vi "datosLecturaQR_to_Arduino.vi"(8 "error in (no error)":errorcluster, 9 "LECTURA QR INPUT":T1={"COORD X"=0, "COORD  Y"=0, "NºASICS"=1, "SELECCIÓN DE BANDEJA"=enum."BANDEJA ENTRADA", "CONTEO QR"=0}, 11 "VISA resource name":refnum<visa-resource-name>) -> (0 "error IO":errorcluster, 2 "celda de comienzo leída":string)   [LabVIEW 2019]
uses:
  TYPE'S DEF/INPUT LECTURA_QR.ctl
  <vilib>/Utility/error.llb/Error Cluster From Error Code.vi
  <vilib>/ErrorRing/Error Ring.xnode
panel:
  out "trama datos":string
  # "CELDA DE COMIENZO"
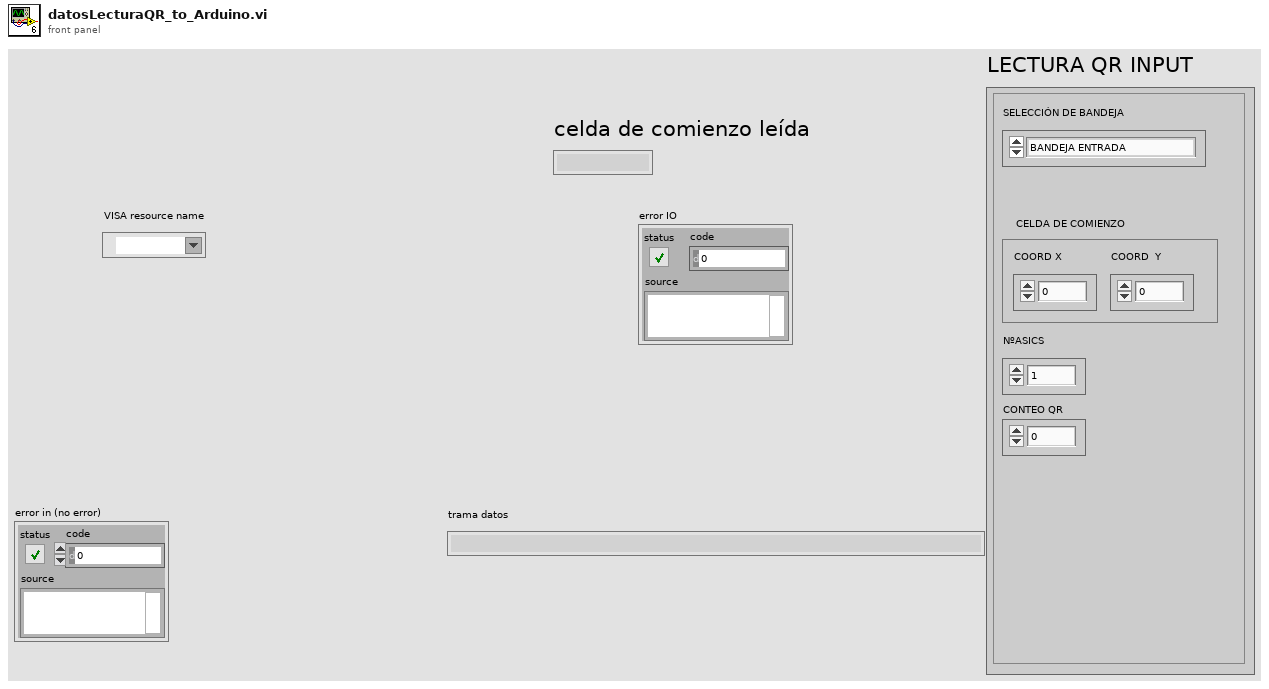
[diagram p1: front panel]
types:
  T1 = typedef "INPUT LECTURA_QR.ctl" = cluster{"COORD X":u16, "COORD  Y":u16, "NºASICS":u32, "SELECCIÓN DE BANDEJA":enum16{"BANDEJA ENTRADA", "BANDEJA OK", "BANDEJA NOK"}, "CONTEO QR":u32}
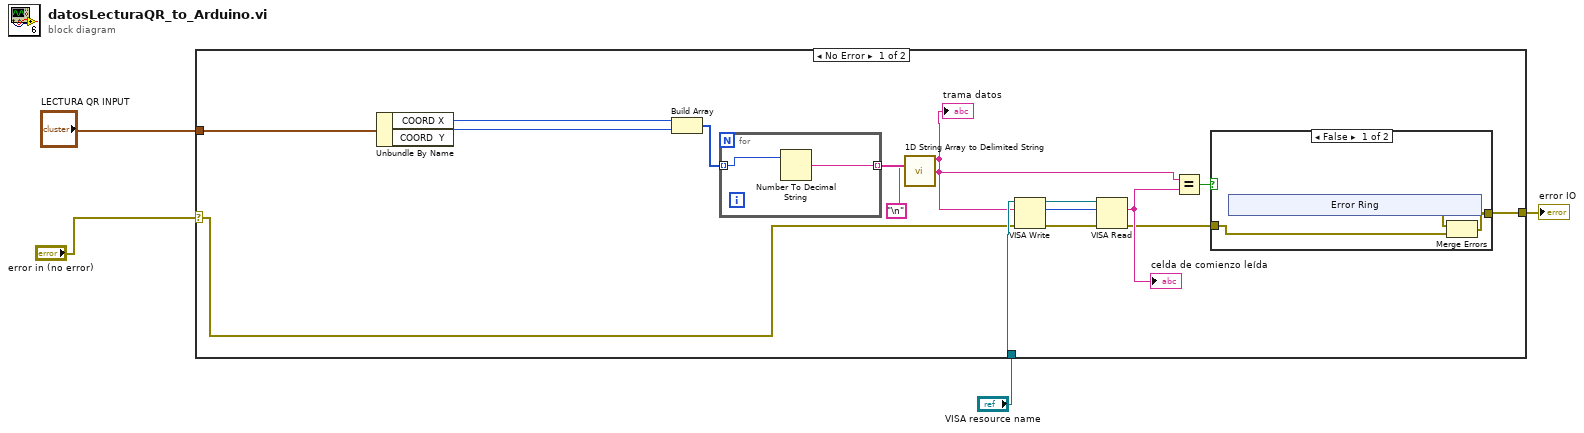
[diagram p0: block diagram]
diagram:
  n1 = case shown="No Error" "error in (no error)" {
    selector: "error in (no error)" -> [w16 w32]
    tunnel: "VISA resource name" -> [w17 _]
    tunnel: [w9 w32] -> w2
    tunnel: "LECTURA QR INPUT" -> [w5 _]
    frame No Error {
      n2 = Unbundle By Name(w5) -> ("COORD X"=w7:u16, "COORD  Y"=w6:u16)
      n3 = Build Array(w7, w6) -> (w20:u16[])
      n4 = for {
        tunnel: w20 -> [w30] mode=indexing
        tunnel: [w31] -> w19 mode=indexing
        n5 = Number To Decimal String(number=w30) -> (decimal integer string=w31:string)  [unwired: 1 in]
      }
      n6 = call <vilib>:"1D String Array to Delimited String.vi"("delimiter"="\n", "string array"=w19) -> ("delimited string"=w12:string)  [unwired: 9 in]
      "trama datos" <- w12
      n7 = VISA Write(VISA resource name=w17, write buffer=w12, error in (no error)=w16) -> (VISA resource name out=w14:refnum<visa-resource-name>, return count=w13:u32, error out=w15:errorcluster)
      n8 = VISA Read(VISA resource name=w14, byte count=w13, error in (no error)=w15) -> (read buffer=w11:string, error out=w8:errorcluster)  [unwired: 2 out]
      "celda de comienzo leída" <- w11
      n9 = Equal?(x=w12, y=w11) -> (x = y?=w10:bool)
      n10 = case shown="False" w10 {
        tunnel: [w23 w29] -> w9
        tunnel: w8 -> [w21 w29]
        frame False {
          n11 = xnode "Error Ring"() -> ("error out"=w22:errorcluster)
          n12 = Merge Errors(w22, w21) -> (w23:errorcluster)
        }
        frame True {
        }
      }
    }
    frame Error {
    }
  }
  "error IO" <- w2
